vi "Global_SM to HW Data.vi"() -> ()   [LabVIEW 2017, in "Intake.lvlib"]
uses:
  Intake.lvlib
panel:
  in  "SM_Intake_HW Speed":dbl
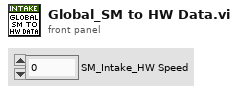
[diagram p1: front panel]
diagram:
